vi "Read Multiplier.vi"(8 "error in (no error)":errorcluster, 11 "Encryption in":refnum<class "Encryption.lvclass">) -> (0 "error out":errorcluster, 2 "Multiplier":dbl, 3 "Encryption out":refnum<class "Encryption.lvclass">)   [LabVIEW 2019, in "TSC Event Logger.lvlib" / "Encryption.lvclass"]
doc: "Data Member Access method to read the multiplier on the object.\n\n<b>Code Developed By:</b>\nTechnology Service Corporation\nBloomington, IN 47403\nwww.tsc.com/atcs\n\nDeveloper:\nDaniel Coons"
uses:
  Encryption.lvclass
  Encryption.lvclass/Encryption.ctl
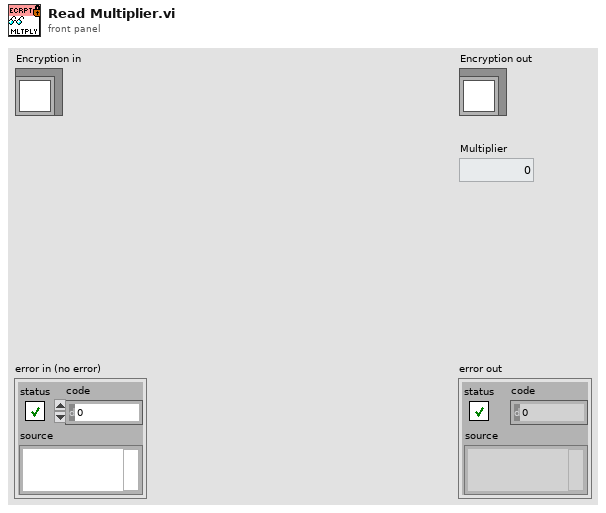
[diagram p1: front panel]
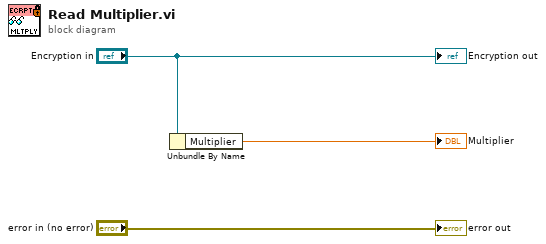
[diagram p0: block diagram]
diagram:
  n1 = Unbundle By Name("Encryption in") -> ("Multiplier"=→"Multiplier":dbl)
  "error out" <- "error in (no error)"
  "Encryption out" <- "Encryption in"
